vi "About this VI.vi"(8 "Error In":errorcluster) -> (0 "Error Out":errorcluster)   [LabVIEW 2015]
doc: "This VI Provides the user with information about the program."
panel:
  in  "OK Button":bool
  # "About myRoboLab"
  # "The simulation in this project is part of my placement years project.\nmyRoboLab is aimed for students and Robot enthusiasts who would like to \nlearn the basics about robotic arms in a fun and interactive way.\nThe three-degree of freedom robotic arm seen on the right is custom made, \ndesigned especially for this project. As the robotic arm has three degrees of \nfreedom, it means that with the use of three servo motors it is able to move in \na three dimensional space. Furthermore, with the use of an extra motor at the \nclamp it is also able to pick up objects. \nAs not everyone will have access to the robotic arm, a simulation is also \ndisplayed on the screen moving in the exact same manner as the robotic arm in \norder to increase the amount of people who can benefit from this project.\nThis project was designed as part of my individual placement year project in \norder to help everyone with a huge passion for robotics, like myself, learn as \nmuch as they can about it in a fun way. \nIf you would like to ask me any questions regarding the project or would like \nto give me feedback please feel free to do so at the community page where you \ncan find more details about the project as well as all the designs of the robotic \narm."
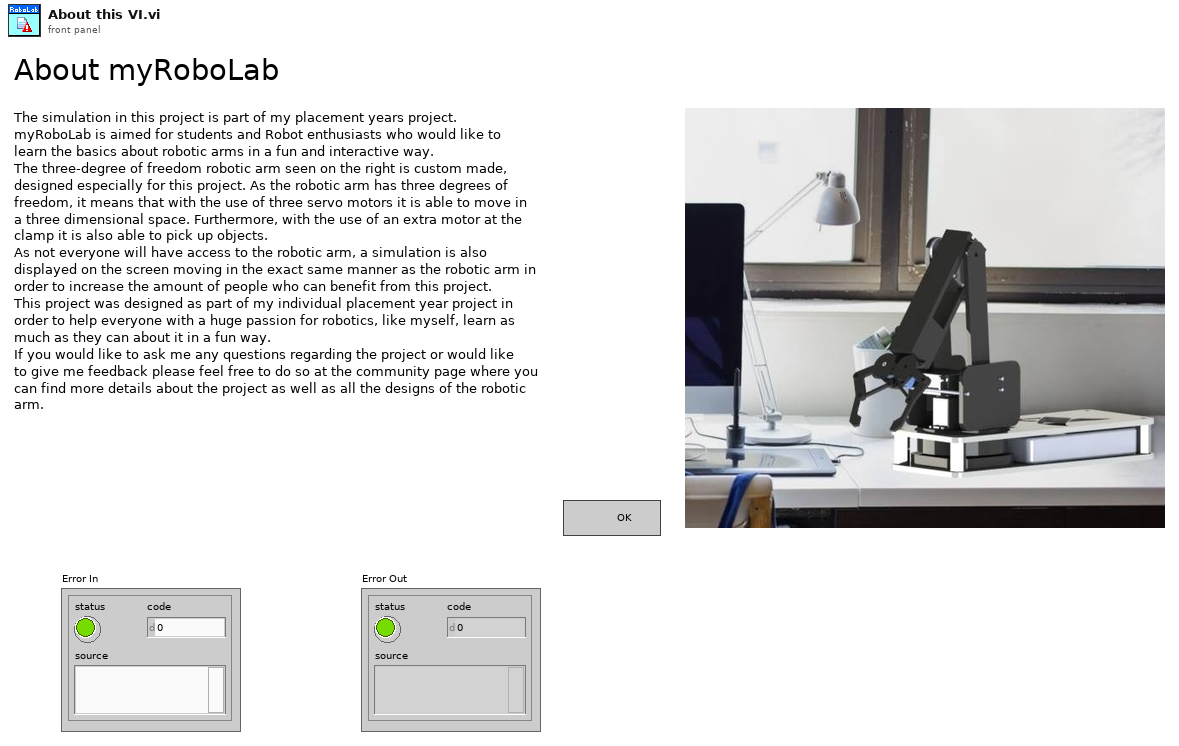
[diagram p1: front panel]
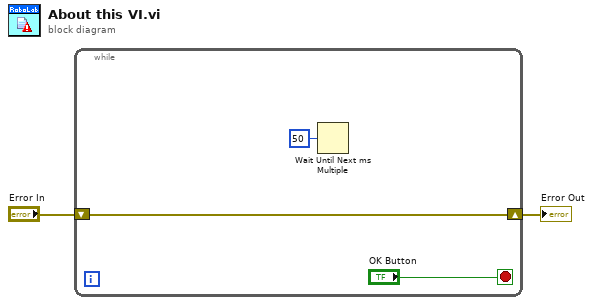
[diagram p0: block diagram]
diagram:
  n1 = while {
    shift-right: [w3] -> w1
    shift-left: "Error In" -> [w3]
    stop <- "OK Button" stop-if-true
    n2 = Wait Until Next ms Multiple(millisecond multiple=u32 50) -> ()  [unwired: 1 out]
  }
  "Error Out" <- w1
